vi "close wrapper.vi"(8 "error in (no error)":errorcluster, 11 "module in":refnum<class "TBM module execution interface.lvclass">) -> (0 "error out":errorcluster)   [LabVIEW 2013, in "TBM module execution interface.lvclass"]
uses:
  TBM module execution interface.lvclass
  <vilib>/NI/Syslog Wrapper - Linux/write syslog.vi
  <vilib>/Utility/LVClass/Get LV Class Name.vi
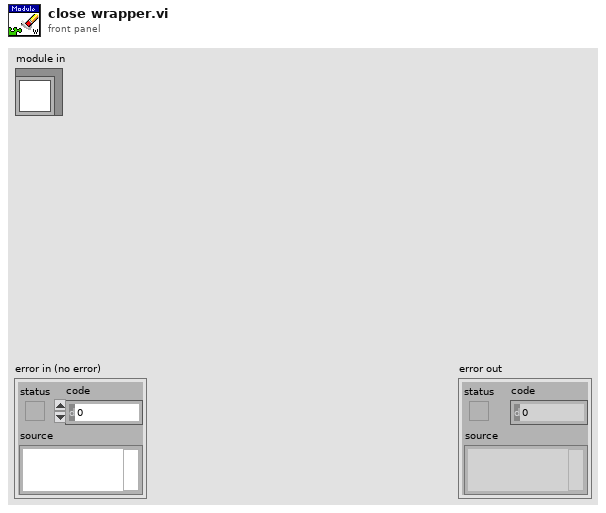
[diagram p1: front panel]
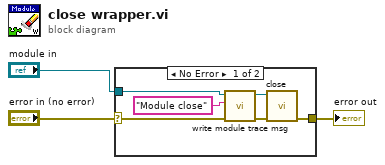
[diagram p0: block diagram]
diagram:
  n1 = case shown="No Error" "error in (no error)" {
    selector: "error in (no error)" -> [w7 w10]
    tunnel: [w4 w10] -> w2
    tunnel: "module in" -> [w8 _]
    frame No Error {
      n2 = call "write module trace msg.vi"("error in (no error)"=w7, "message"="Module close", "module in"=w8) -> ("error out"=w6:errorcluster, "module out"=w9:refnum<class "TBM module execution interface.lvclass">)  [unwired: 7 in]
      n3 = call-dynamic "close.vi"("error in"=w6, "module in"=w9) -> ("error out"=w4:errorcluster)  [unwired: 9 in]
    }
    frame Error {
    }
  }
  "error out" <- w2
